vi "InverseImg.vi"(0 "MirrorAxis (0=y, 1=x)":i32, 1 "Array":sgl[][](array[numeric])) -> (3 "InvertedImg":sgl[][](array[numeric]))   [LabVIEW 2019]
uses:
  <vilib>/Analysis/Matrix/Datatypes/RealMatrix.ctl
  <vilib>/Analysis/Matrix/Numeric/Conversions/Array To Matrix - RA2.vi
  <vilib>/Analysis/Matrix/Numeric/Multiply/Multiply - RM,RM.vi
  <vilib>/Analysis/Matrix/NI_Matrix.lvlib
panel:
  out "A * B":T1
  in  "Astrometry OUT":T2
  in  "Astrometry IN":T2
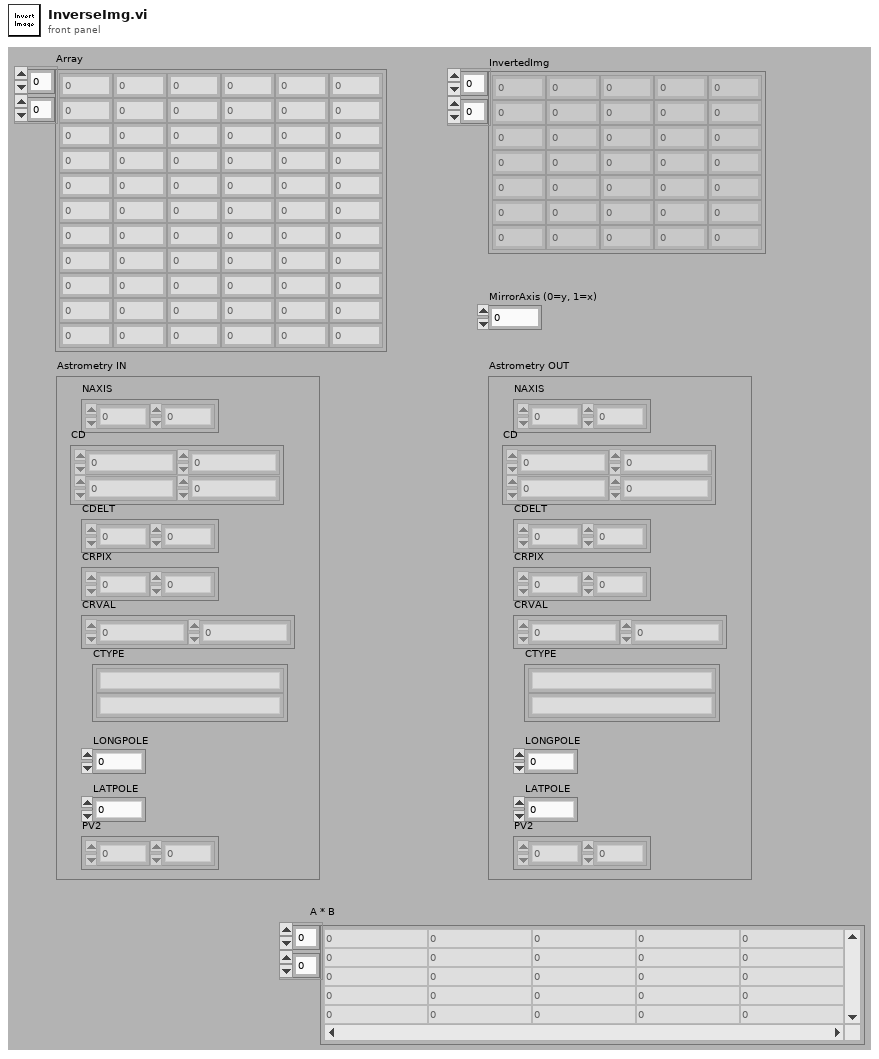
[diagram p1: front panel]
types:
  T1 = typedef "NI_Matrix.lvlib/RealMatrix.ctl" = dbl[][]
  T2 = cluster{"NAXIS":dbl[], "CD":dbl[][], "CDELT":dbl[], "CRPIX":dbl[], "CTYPE":string[], "CRVAL":dbl[], "LONGPOLE":dbl, "LATPOLE":dbl, "PV2":dbl[]}
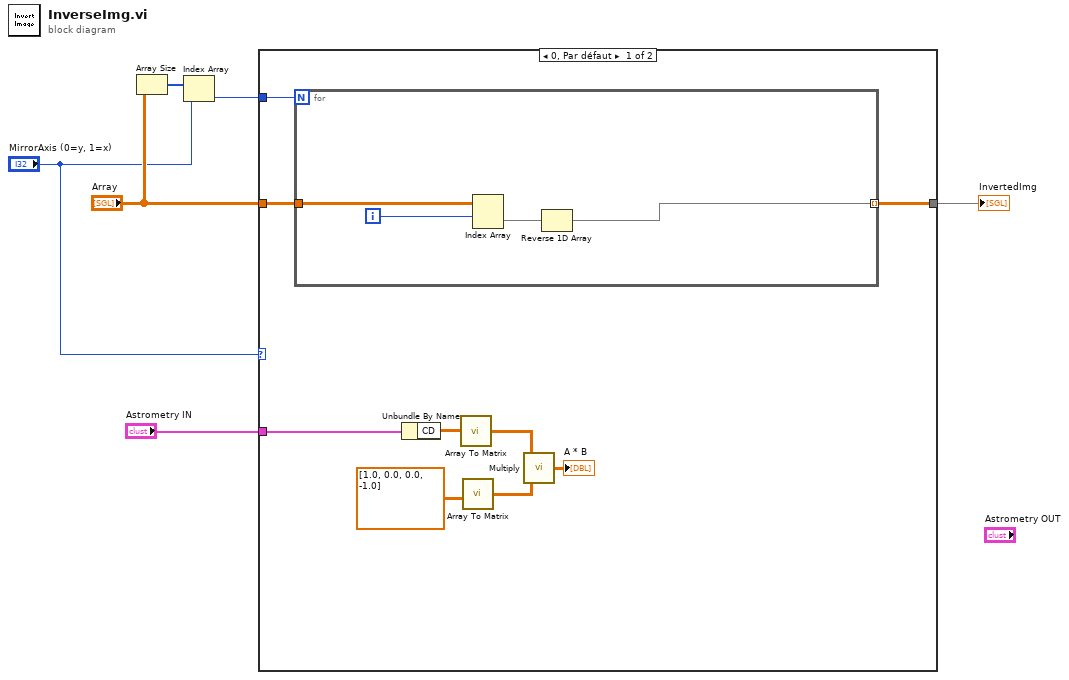
[diagram p0: block diagram]
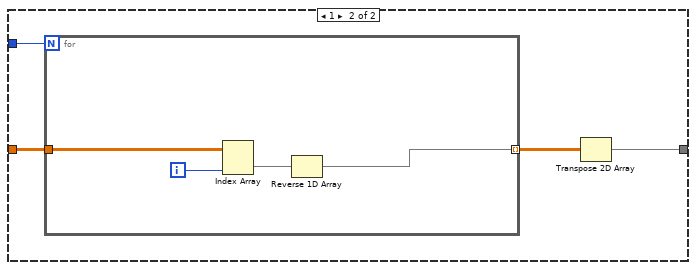
[diagram p2: hidden frame]
diagram:
  n1 = Array Size(array="Array") -> (size(s)=w6:i32[])
  n2 = Index Array(array=w6, index="MirrorAxis (0=y, 1=x)") -> (element=w4:i32)
  n3 = case shown="0, Par défaut" "MirrorAxis (0=y, 1=x)" {
    tunnel: "Array" -> [w15 w23]
    tunnel: w4 -> [w14 w22]
    tunnel: [w13 w20] -> w2
    tunnel: "Astrometry IN" -> [w12 _]
    frame 0, Default {
      n4 = for {
        N: w14 -> [_]
        tunnel: w15 -> [w18]
        tunnel: [w17] -> w13 mode=indexing
        i -> [w16]
        n5 = Index Array(array=w18, index (row)=w16) -> (element=w19:sgl[])  [unwired: 1 in]
        n6 = Reverse 1D Array(array=w19) -> (reversed array=w17:sgl[])
      }
      n7 = Unbundle By Name(w12) -> ("CD"=w10:dbl[][])
      n8 = call-poly <vilib>:"Array To Matrix.vi"("Real 2D Array"=w10) -> ("Real Matrix"=w9:T1)
      n9 = call-poly <vilib>:"Array To Matrix.vi"("Real 2D Array"=dbl[][] [[1.0, 0.0], [0.0, -1.0]]) -> ("Real Matrix"=w8:T1)
      n10 = call-poly <vilib>:"Multiply.vi"("Real Matrix B"=w8, "Real Matrix A"=w9) -> ("A * B"=→"A * B":T1)
    }
    frame 1 {
      n11 = for {
        N: w22 -> [_]
        tunnel: w23 -> [w26]
        tunnel: [w25] -> w21 mode=indexing
        i -> [w24]
        n12 = Index Array(array=w26, index (col)=w24) -> (element=w27:sgl[])  [unwired: 1 in]
        n13 = Reverse 1D Array(array=w27) -> (reversed array=w25:sgl[])
      }
      n14 = Transpose 2D Array(2D array=w21) -> (transposed array=w20:sgl[][])
    }
  }
  "InvertedImg" <- w2
